vi "Ritter Wet Meter Calculations.vi"(0 "Heise Barometric Pressure (inHG)":dbl, 1 "Gas Pressure (in WC)":dbl, 3 "Gas Flow Rate (cuft/hr)-Uncorrected":dbl, 4 "Totalized Flow (cuft)-Uncorrected":dbl, 5 "error in (no error)":errorcluster, 6 "Gas Temperature (F)":dbl, 7 "Gross Heating Value, Vol (Real, Sat)":dbl, 8 "standardPressure (in HG)":dbl=30.0) -> (10 "E":dbl, 11 "btuEnergy":dbl, 12 "CFsat":dbl, 13 "btuRate":dbl, 14 "tempCorrectionFactor":dbl, 15 "pressureCorrectionFactor":dbl, 17 "gasFlowRate":dbl, 18 "gasVolume":dbl, 19 "error out":errorcluster)   [LabVIEW 2023]
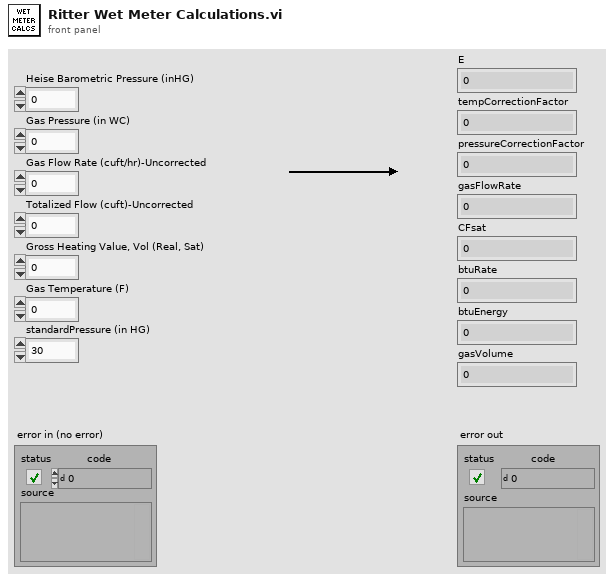
[diagram p1: front panel]
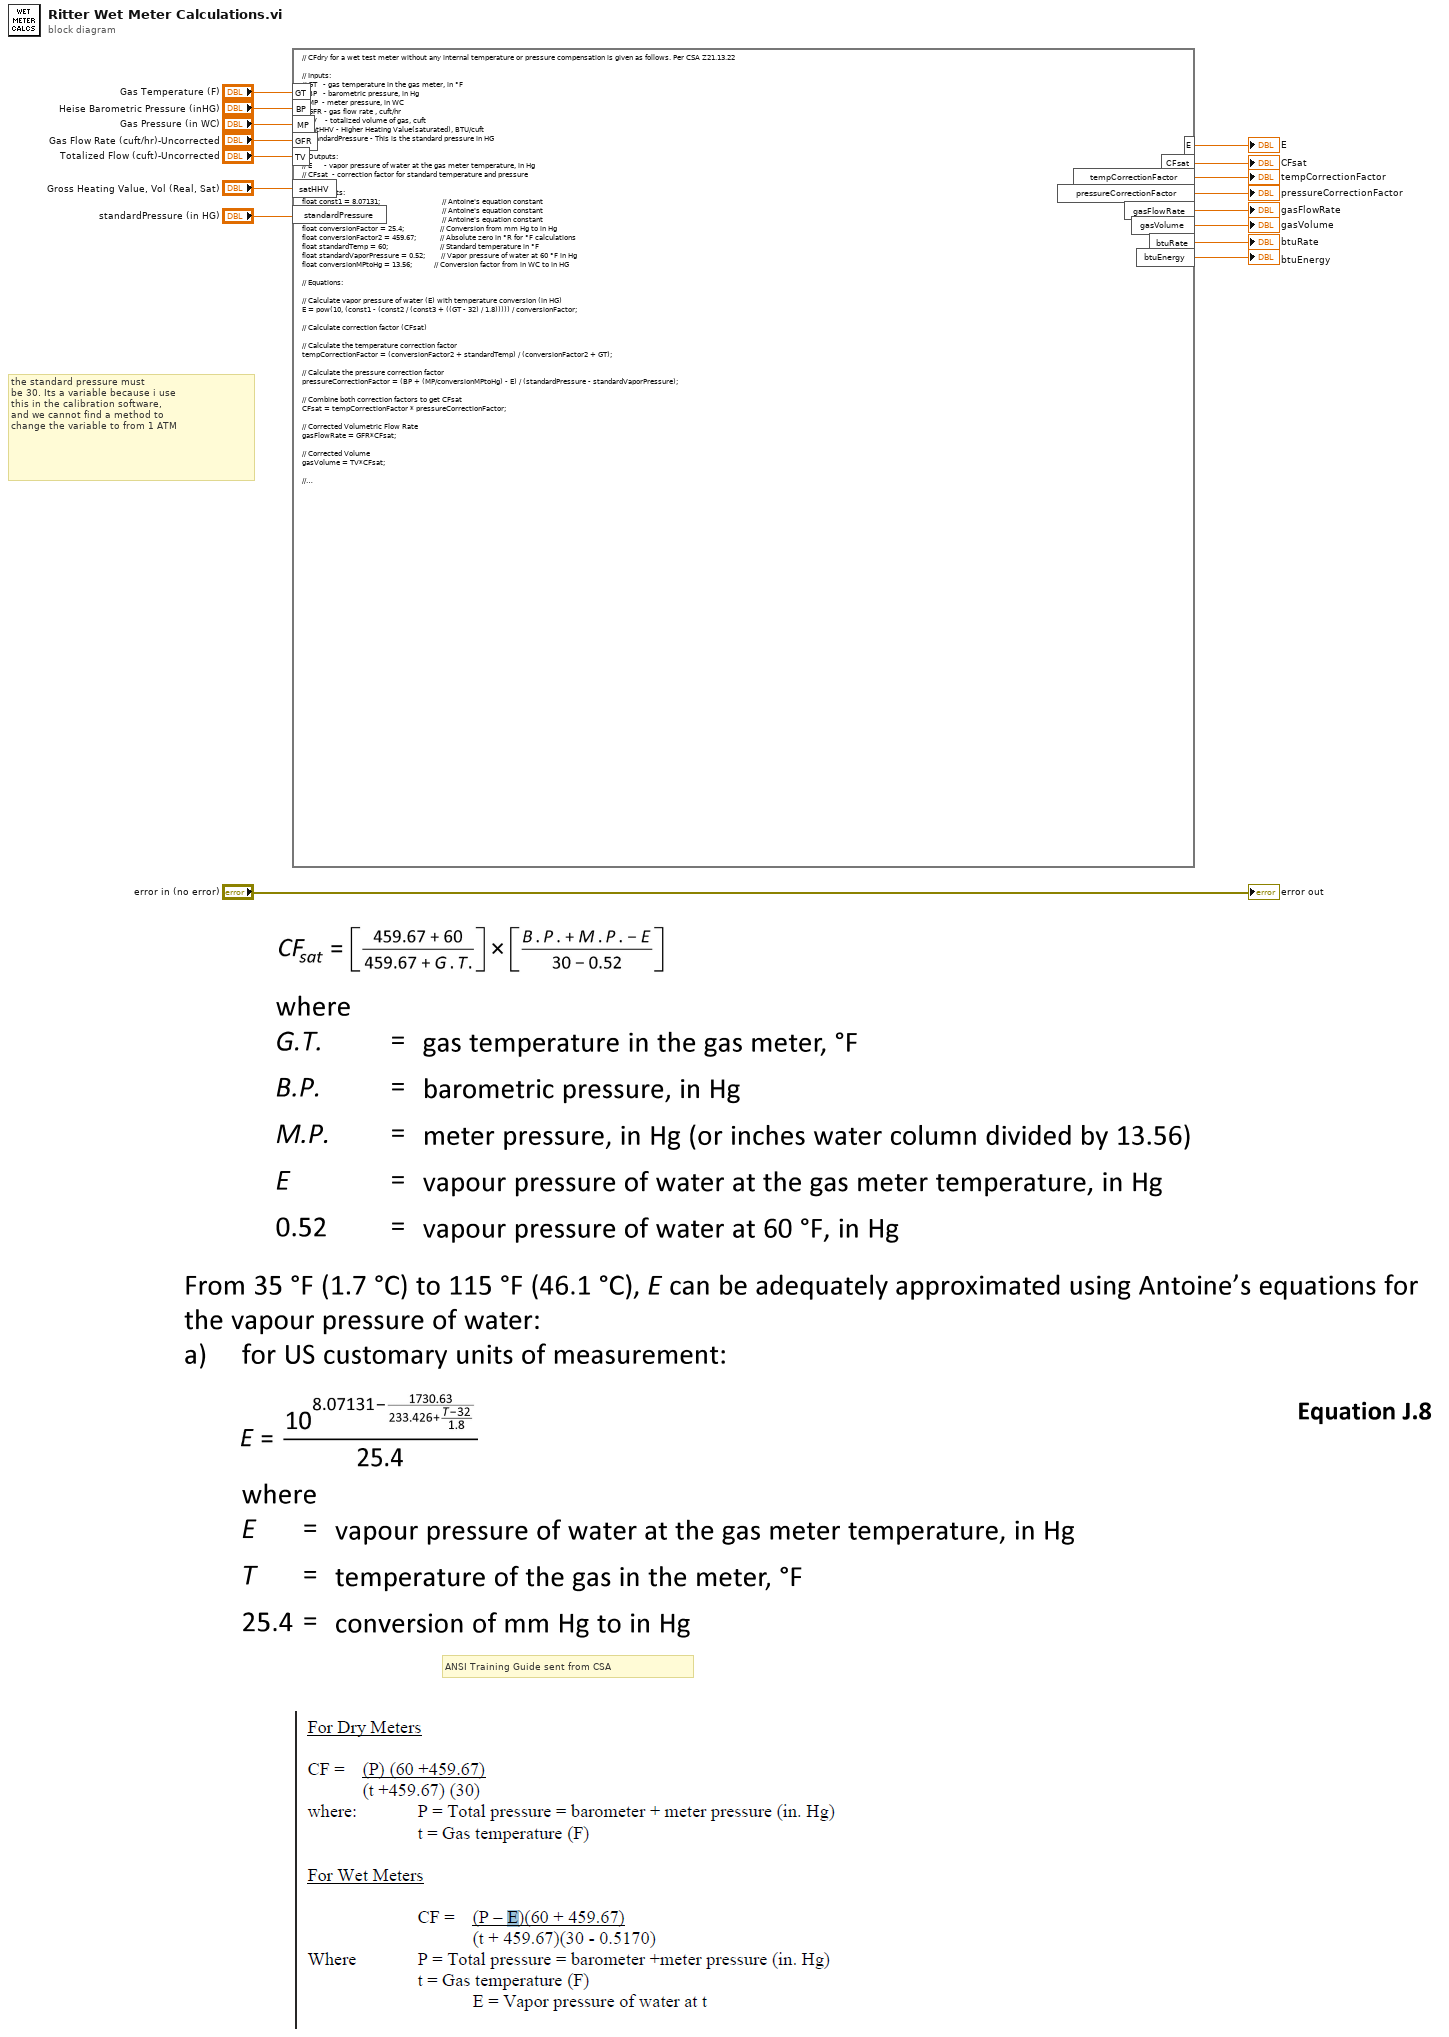
[diagram p0: block diagram]
diagram:
  # "the standard pressure must\nbe 30. Its a variable because i use\nthis in the calibration software, \nand we cannot find a method to\nchange the variable to from 1 ATM"
  # "ANSI Training Guide sent from CSA"
  n1 = formula code="// CFdry for a wet test meter without any internal temperature or pressure compensation is given as follows. Per CSA Z21.13.22  \n\n// Inputs:\n// GT   - gas temperature in the gas meter, in °F\n// BP   - barometric pressure, in Hg\n// MP  - meter pressure, in WC\n// GFR - gas flow rate , cuft/hr\n// TV    - totalized volume of gas, cuft\n// satHHV - Higher Heating Value(saturated), BTU/cuft\n// standardPressure - This is the standard pressure in HG\n\n// Outputs:\n// E      - vapor pressure of water at the gas meter temperature, in Hg\n// CFsat  - correction factor for standard temperature and pressure\n\n// Constants:\nfloat const1 = 8.07131;                               // Antoine's equation constant\nfloat const2 = 1730.63;                               // Antoine's equation constant\nfloat const3 = 233.426;                               // Antoine's equation constant\nfloat conversionFactor = 25.4;                  // Conversion from mm Hg to in Hg\nfloat conversionFactor2 = 459.67;            // Absolute zero in °R for °F calculations\nfloat standardTemp = 60;                          // Standard temperature in °F\nfloat standardVaporPressure = 0.52;        // Vapor pressure of water at 60 °F in Hg\nfloat conversionMPtoHg = 13.56;           // Conversion factor from in WC to in HG\n\n// Equations:\n\n// Calculate vapor pressure of water (E) with temperature conversion (in HG)\nE = pow(10, (const1 - (const2 / (const3 + ((GT - 32) / 1.8))))) / conversionFactor;\n\n// Calculate correction factor (CFsat)\n\n// Calculate the temperature correction factor\ntempCorrectionFactor = (conversionFactor2 + standardTemp) / (conversionFactor2 + GT);\n\n// Calculate the pressure correction factor\npressureCorrectionFactor = (BP + (MP/conversionMPtoHg) - E) / (standardPressure - standardVaporPressure);\n\n// Combine both correction factors to get CFsat\nCFsat = tempCorrectionFactor * pressureCorrectionFactor;\n\n// Corrected Volumetric Flow Rate\ngasFlowRate = GFR*CFsat;\n\n// Corrected Volume\ngasVolume = TV*CFsat;\n\n// Rate in BTU/HR\nbtuRate = gasFlowRate*satHHV;\n\n// Energy Usage in BTU\nbtuEnergy=gasVolume*satHHV;"("GT"="Gas Temperature (F)", "BP"="Heise Barometric Pressure (inHG)", "MP"="Gas Pressure (in WC)", "GFR"="Gas Flow Rate (cuft/hr)-Uncorrected", "TV"="Totalized Flow (cuft)-Uncorrected", "satHHV"="Gross Heating Value, Vol (Real, Sat)", "standardPressure"="standardPressure (in HG)") -> ("E"=→"E":dbl, "CFsat"=→"CFsat":dbl, "tempCorrectionFactor"=→"tempCorrectionFactor":dbl, "pressureCorrectionFactor"=→"pressureCorrectionFactor":dbl, "gasFlowRate"=→"gasFlowRate":dbl, "gasVolume"=→"gasVolume":dbl, "btuRate"=→"btuRate":dbl, "btuEnergy"=→"btuEnergy":dbl)
  "error out" <- "error in (no error)"
